vi "zc closure log call.vi"(8 "error in (no error)":errorcluster, 9 "msg":cluster{}, 10 "severity":u32(ring) items=["ZC_LOG_SEVERITY_TRACE", "ZC_LOG_SEVERITY_DEBUG", "ZC_LOG_SEVERITY_INFO", "ZC_LOG_SEVERITY_WARN", "ZC_LOG_SEVERITY_ERROR"], 11 "closure":cluster{}) -> (0 "error out":errorcluster)   [LabVIEW 2021, in "zenohc.lvlib"]
doc: "void zc_closure_log_call(const struct zc_loaned_closure_log_t *closure,\n enum zc_log_severity_t severity,\n const struct z_loaned_string_t *msg);"
uses:
  zenohc.lvlib
  zenohc.dll
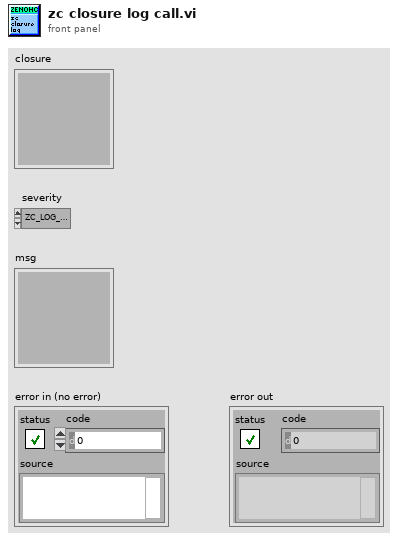
[diagram p1: front panel]
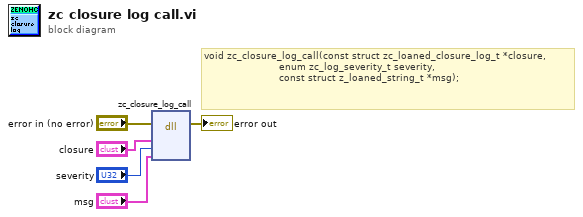
[diagram p0: block diagram]
diagram:
  # "void zc_closure_log_call(const struct zc_loaned_closure_log_t *closure,\n                         enum zc_log_severity_t severity,\n                         const struct z_loaned_string_t *msg);"
  n1 = dll-call lib="D:/dev/zenoh_labview/zenohc/zenohc.*" fn="zc_closure_log_call"(error in="error in (no error)", "closure"="closure", "severity"="severity", "msg"="msg") -> (error out=→"error out":errorcluster)  [unwired: 6 in, 1 out]
